vi "Table Color Init-Reset.vi"(11 "Test Table":refnum<vi>) -> ()   [LabVIEW 2018]
uses:
  <vilib>/Utility/miscctls.llb/LVRowAndColumnTypeDef.ctl
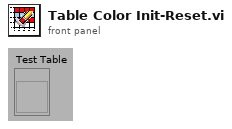
[diagram p1: front panel]
types:
  T1 = typedef "LVRowAndColumnTypeDef.ctl" = cluster{"Row":i32, "Column":i32}
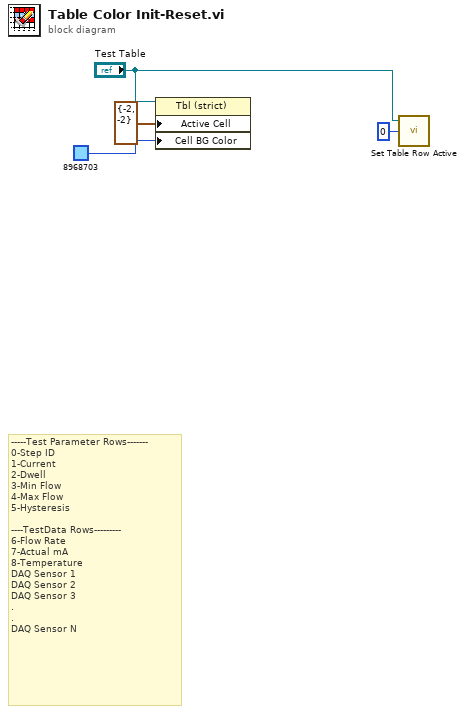
[diagram p0: block diagram]
diagram:
  # "-----Test Parameter Rows-------\n0-Step ID\n1-Current\n2-Dwell\n3-Min Flow\n4-Max Flow\n5-Hysteresis\n\n----TestData Rows---------\n6-Flow Rate\n7-Actual mA\n8-Temperature\nDAQ Sensor 1\nDAQ Sensor 2\nDAQ Sensor 3\n.\n.\nDAQ Sensor N"
  n1 = property class="Tbl (strict)"(reference="Test Table", "Active Cell"=T1 {"Row"=-2, "Column"=-2} ("Active Cell:Active Cell"), "Cell BG Color"=u32 8968703 ("Color Box")) -> ()  [unwired: 1 in, 2 out]
  n2 = call "Set Table Row Active.vi"("Current Step ID"=0, "Test Table"="Test Table") -> ()  [unwired: 1 in]
